vi "Set Values by Primary Key.vi"(8 "error in (no error)":errorcluster, 10 "Primary Key Value":string, 11 "Table in":refnum<class "Table.lvclass">) -> (0 "error out":errorcluster, 3 "Table out":refnum<class "Table.lvclass">)   [LabVIEW 2020, in "Table.lvlib" / "Table.lvclass"]
uses:
  Table.lvclass
  Table.lvclass/Table.ctl
  Table Configuration Interface/Table Configuration Interface.lvclass
  Column Interface/Column Interface Class/Column Interface.lvclass
  Database Interfaces/Database Interface Class/Database Interface.lvclass
panel:
  # "Use this VI to set the value of ALL columns in a table by PK.\nTo set individual columns, use column PK methods."
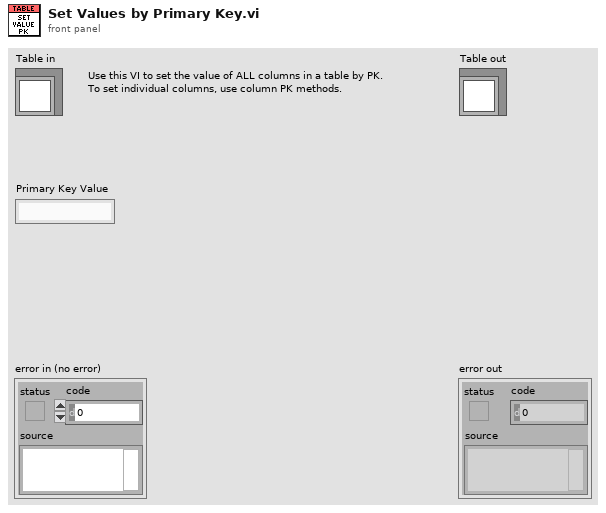
[diagram p1: front panel]
types:
  T1 = map{string, refnum<class "Column Interface.lvclass">}
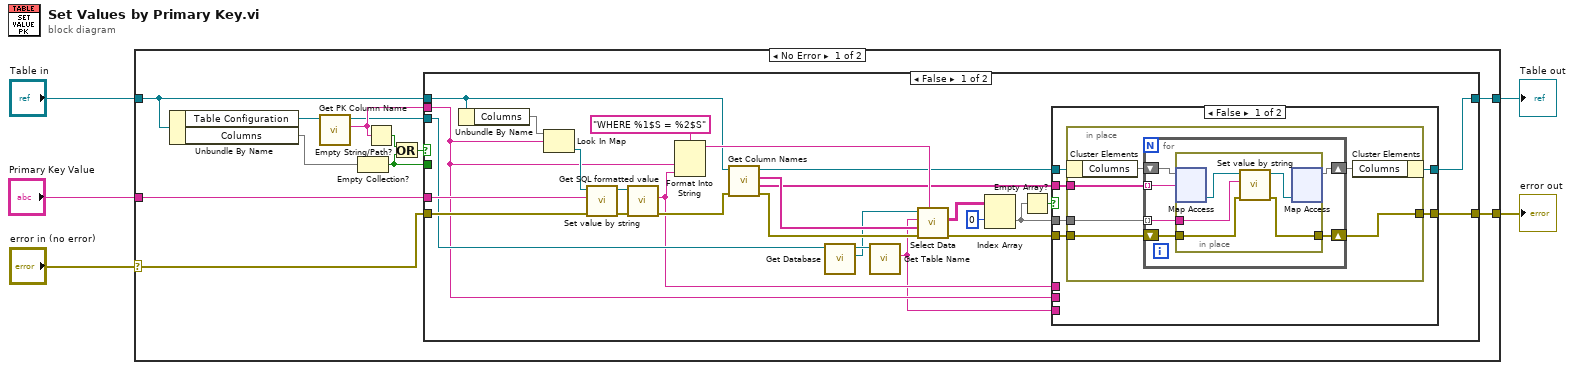
[diagram p0: block diagram]
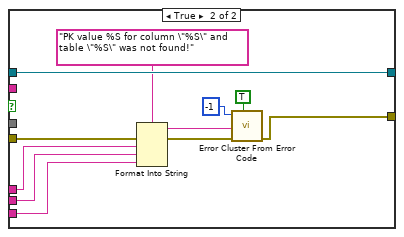
[diagram p2: hidden frame]
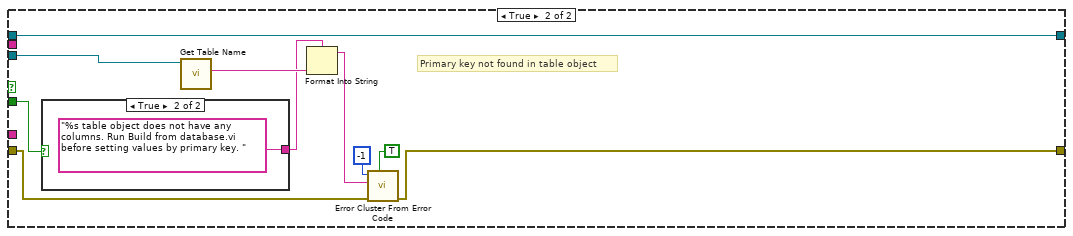
[diagram p3: hidden frame]
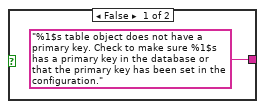
[diagram p4: hidden frame]
diagram:
  n1 = case shown="No Error" "error in (no error)" {
    selector: "error in (no error)" -> [w14 w92]
    tunnel: [w13 w92] -> w4
    tunnel: [w9 w91] -> w2
    tunnel: "Table in" -> [w10 w91]
    tunnel: "Primary Key Value" -> [w17 _]
    frame No Error {
      n2 = Unbundle By Name(w10) -> ("Table Configuration"=w8:refnum<class "Table Configuration Interface.lvclass">, "Columns"=w16:T1)
      n3 = call-dynamic "Get PK Column Name.vi"("Table Configuration Interface in"=w8) -> ("PK Name"=w7:string, "Table Configuration Interface out"=w6:refnum<class "Table Configuration Interface.lvclass">)  [unwired: 8 in, 1 out]
      n4 = Empty Collection?(1:w16) -> (0:w12:bool)
      n5 = Empty String/Path?(string/path=w7) -> (empty?=w11:bool)
      n6 = Or(x=w11, y=w12) -> (x .or. y?=w15:bool)
      n7 = case shown="False" w15 {
        tunnel: w17 -> [w36 _]
        tunnel: w7 -> [w20 _]
        tunnel: w14 -> [w35 w85]
        tunnel: [w38 w84] -> w13
        tunnel: w12 -> [_ w88]
        tunnel: w10 -> [w26 w83]
        tunnel: [w27 w83] -> w9
        tunnel: w6 -> [w25 w81]
        frame False {
          n8 = Unbundle By Name(w26) -> ("Columns"=w42:T1)
          n9 = Look In Map(map=w42, key=w20) -> (value=w37:refnum<class "Column Interface.lvclass">)  [unwired: 1 in, 1 out]
          n10 = call-dynamic "Set value by string.vi"("error in (no error)"=w35, "Value"=w36, "Column Interface in"=w37) -> ("error out"=w33:errorcluster, "Column Interface out"=w34:refnum<class "Column Interface.lvclass">)  [unwired: 7 in]
          n11 = call-dynamic "Get SQL formatted value.vi"("error in (no error)"=w33, "Column Interface in"=w34) -> ("error out"=w32:errorcluster, "Formatted Value"=w19:string)  [unwired: 7 in, 1 out]
          n12 = Format Into String(format string="WHERE %1$S = %2$S", w20, w19) -> (resulting string=w43:string)  [unwired: 2 in, 1 out]
          n13 = call "Get Column Names.vi"("error in (no error)"=w32, "Table in"=w26) -> ("error out"=w31:errorcluster, "Key Names"=w29:string[], "Column Names"=w30:string[], "Table out"=w28:refnum<class "Table.lvclass">)  [unwired: 6 in]
          n14 = call-dynamic "Get Database.vi"("Table Configuration Interface in"=w25) -> ("Database"=w23:refnum<class "Database Interface.lvclass">, "Table Configuration Interface out"=w24:refnum<class "Table Configuration Interface.lvclass">)  [unwired: 8 in, 1 out]
          n15 = call-dynamic "Get Table Name.vi"("Table Configuration Interface in"=w24) -> ("Table Name"=w18:string)  [unwired: 8 in, 2 out]
          n16 = call-dynamic "Select Data.vi"("WHERE Statement"=w43, "error in (no error)"=w31, "Columns"=w30, "Table"=w18, "Database Interface in"=w23) -> ("error out"=w39:errorcluster, "Data"=w41:string[][])  [unwired: 4 in, 1 out]
          n17 = Index Array(array=w41, index (row)=0) -> (element=w21:string[])  [unwired: 1 in]
          n18 = Empty Array?(array=w21) -> (empty?=w22:bool)
          n19 = case shown="False" w22 {
            tunnel: w39 -> [w50 w76]
            tunnel: [w49 w68] -> w38
            tunnel: w29 -> [w48 _]
            tunnel: w28 -> [w47 w78]
            tunnel: [w46 w78] -> w27
            tunnel: w21 -> [w45 _]
            tunnel: w20 -> [_ w74]
            tunnel: w19 -> [_ w75]
            tunnel: w18 -> [_ w73]
            frame False {
              n20 = in-place {
                in-place-border: w50 -> [w56]
                in-place-border: [w55] -> w49
                in-place-border: w48 -> [w54]
                in-place-border: w45 -> [w51]
                n21 = in-place-cluster #1(w47) -> ("Columns"=w53:T1)
                n22 = for {
                  tunnel: w54 -> [w62] mode=indexing
                  shift-right: [w60] -> w52
                  shift-left: w53 -> [w61]
                  shift-right: [w58] -> w55
                  shift-left: w56 -> [w59]
                  tunnel: w51 -> [w57] mode=indexing
                  n23 = in-place {
                    in-place-border: w59 -> [w65]
                    in-place-border: [w64] -> w58
                    in-place-border: w57 -> [w63]
                    n24 = in-place-map #2(w61, w62) -> (w67:refnum<class "Column Interface.lvclass">)  [unwired: 1 in, 1 out]
                    n25 = call-dynamic "Set value by string.vi"("error in (no error)"=w65, "Value"=w63, "Column Interface in"=w67) -> ("error out"=w64:errorcluster, "Column Interface out"=w66:refnum<class "Column Interface.lvclass">)  [unwired: 7 in]
                    n26 = in-place-map #2(w66) -> (w60:T1)  [unwired: 1 in, 2 out]
                  }
                }
                n27 = in-place-cluster #1("Columns"=w52) -> (w46:refnum<class "Table.lvclass">)
              }
            }
            frame True {
              n28 = Format Into String(format string="PK value %S for column \"%S\" and table \"%S\" was not found!", error in=w76, w75, w74, w73) -> (resulting string=w72:string, error out=w69:errorcluster)  [unwired: 1 in]
              n29 = call <vilib>:"Error Cluster From Error Code.vi"("show call chain? (False)"=TRUE, "error in (no error)"=w69, "error message (\"\")"=w72, "error code (0)"=-1) -> ("error out"=w68:errorcluster)  [unwired: 5 in]
            }
          }
        }
        frame True {
          # "Primary key not found in table object"
          n30 = case shown="True" w88 {
            tunnel: ["%1$s table object does not have a primary key. Check to make sure %1$s has a primary key in the database or that the primary key has been set in the configuration." "%s table object does not have any columns. Run Build from database.vi before setting values by primary key. "] -> w79
            frame False {
            }
            frame True {
            }
          }
          n31 = call-dynamic "Get Table Name.vi"("Table Configuration Interface in"=w81) -> ("Table Name"=w82:string)  [unwired: 8 in, 2 out]
          n32 = Format Into String(format string=w79, w82) -> (resulting string=w80:string)  [unwired: 2 in, 1 out]
          n33 = call <vilib>:"Error Cluster From Error Code.vi"("show call chain? (False)"=TRUE, "error in (no error)"=w85, "error message (\"\")"=w80, "error code (0)"=-1) -> ("error out"=w84:errorcluster)  [unwired: 5 in]
        }
      }
    }
    frame Error {
    }
  }
  "error out" <- w4
  "Table out" <- w2
